vi "GameMode.vi"(11 "DataIn":T5) -> (3 "DataOut":T1)   [LabVIEW 2017]
doc: "SubVI criada para mostrar um pop up para o usuário no caso de jogo multiplayer. O usuário poderá escolher entre as opções Um computador, em que os dois jogadores utilizam a mesma máquina, ou Pela Rede, em que cada computador joga por uma máquina."
uses:
  controls/DataIn.ctl
  controls/Tabuleiro.ctl
  controls/GameOption.ctl
  controls/GameMode.ctl
  controls/DataOut.ctl
panel:
  in  "Rede":bool
  in  "Computador":bool
  # "Qual modo de jogo?"
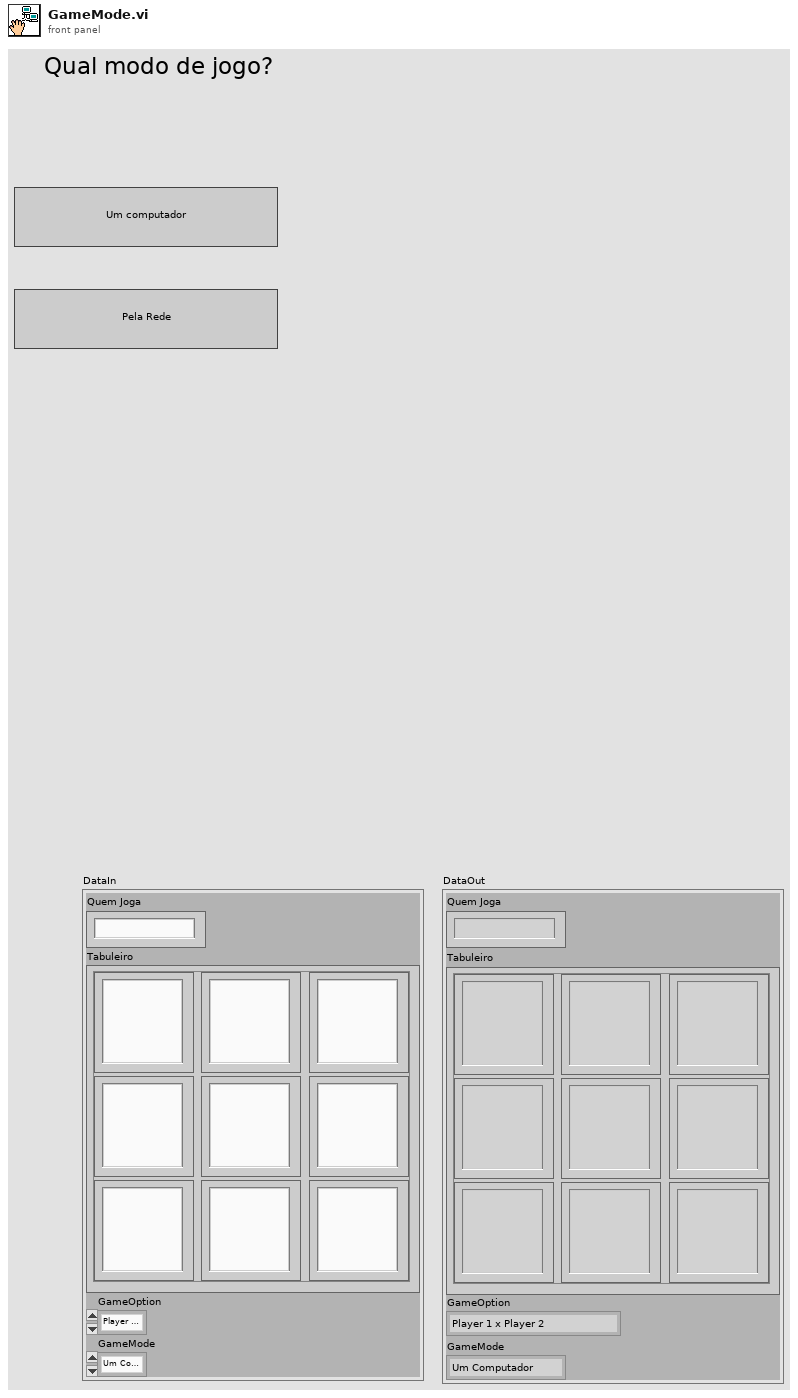
[diagram p1: front panel]
types:
  T1 = typedef "DataOut.ctl" = cluster{"Quem Joga":string, "Tabuleiro":T2, "GameOption":T3, "GameMode":T4}
  T2 = typedef "Tabuleiro.ctl" = cluster{"(0,0)":string, "(1,0)":string, "(0,1)":string, "(1,1)":string, "(2,0)":string, "(1,2)":string, "(2,2)":string, "(0,2)":string, "(2,1) ":string}
  T3 = typedef "GameOption.ctl" = enum16{"Player 1 x Player 2", "Player 1 x Computador"}
  T4 = typedef "GameMode.ctl" = enum16{"Um Computador", "Pela Rede"}
  T5 = typedef "DataIn.ctl" = cluster{"Quem Joga":string, "Tabuleiro":T2, "GameOption":T3, "GameMode":T4}
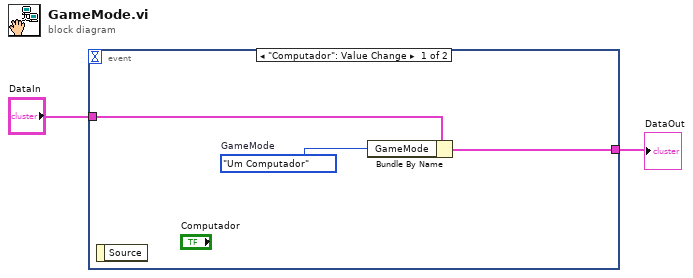
[diagram p0: block diagram]
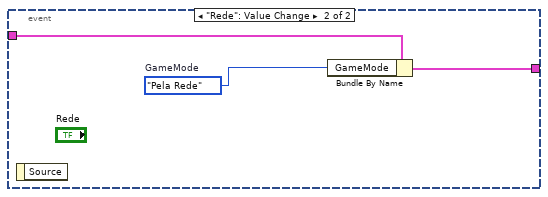
[diagram p2: hidden frame]
diagram:
  n1 = event shown="[0] \"Computador\": Value Change" {
    selector: _ -> [_ _]
    dyn-events: _ -> [_ _]
    timeout: _ -> [_ _]
    tunnel: [w5 w8] -> w2
    tunnel: "DataIn" -> [w4 w7]
    event "Computador": Value Change {
      w3 = GameMode."Um Computador"  # GameMode
      n2 = event-data() -> ()  [unwired: 1 in, 1 out]
      n3 = Bundle By Name(cluster=w4, "GameMode"=w3) -> (w5:T5)
    }
    event "Rede": Value Change {
      w6 = GameMode."Pela Rede"  # GameMode
      n4 = event-data() -> ()  [unwired: 1 in, 1 out]
      n5 = Bundle By Name(cluster=w7, "GameMode"=w6) -> (w8:T5)
    }
  }
  "DataOut" <- w2
